vi "GetSystemInformation.vi"(9 "HighSpeedEServer":refnum<k24>, 11 "error in (no error)":errorcluster) -> (0 "SoftwareVersion":string, 1 "Parameter":string, 2 "Name":string, 3 "error out":errorcluster)   [LabVIEW 2017, in "UnderAutomation.Yaskawa.lvlib"]
uses:
  UnderAutomation.Yaskawa.lvlib
  C:/Users/fg/Documents/Yaskawa.vi/LabVIEW_2024/UnderAutomation.Yaskawa/lib/UnderAutomation.Yaskawa.dll
  LabVIEW_2024/UnderAutomation.Yaskawa/lib/UnderAutomation.Yaskawa.dll
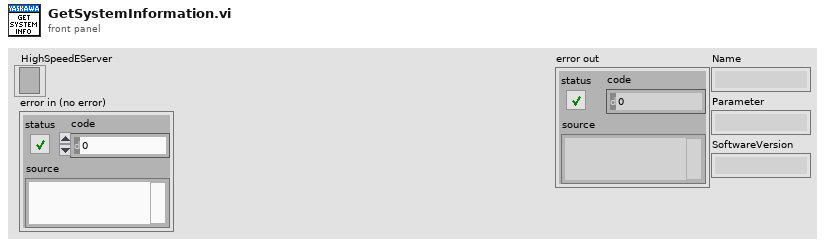
[diagram p1: front panel]
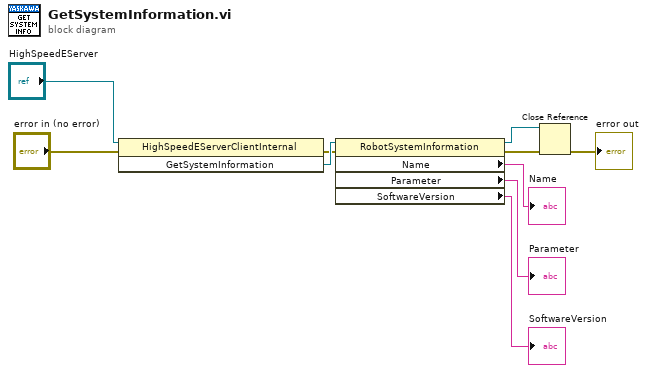
[diagram p0: block diagram]
diagram:
  n1 = invoke class="HighSpeedEServerClientInternal" method="GetSystemInformation"(reference="HighSpeedEServer", error in="error in (no error)") -> (error out=w7:errorcluster, "GetSystemInformation"=w8:refnum<k24>)  [unwired: 1 in, 1 out]
  n2 = property class="RobotSystemInformation"(reference=w8, error in=w7) -> (reference out=w1:refnum<k24>, error out=w3:errorcluster, "Name"=→"Name":string, "Parameter"=→"Parameter":string, "SoftwareVersion"=→"SoftwareVersion":string)
  n3 = Close Reference(reference=w1, error in (no error)=w3) -> (error out=→"error out":errorcluster)
